vi "Efficiency Math.vi"(4 "SMU 2 Current Measurements":dbl[](array[numeric]), 5 "SMU 1 Voltage Measurements":dbl[](array[numeric]), 6 "SMU 2 Voltage Measurements":dbl[](array[numeric]), 7 "SMU 1 Current Measurements":dbl[](array[numeric]), 9 "# Voltage Divisions":i32, 10 "# Points":i32, 11 "XYGraph in":refnum<vi>) -> (3 "Array":cluster{"Array":dbl[], "Array":dbl[]}[](array[cluster]))   [LabVIEW 2014]
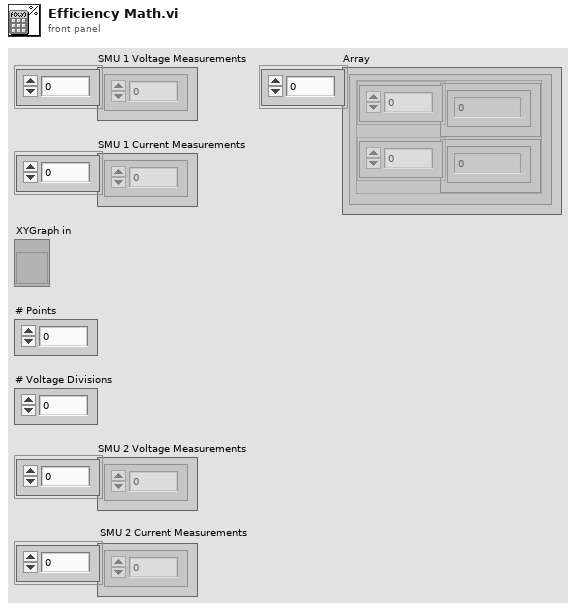
[diagram p1: front panel]
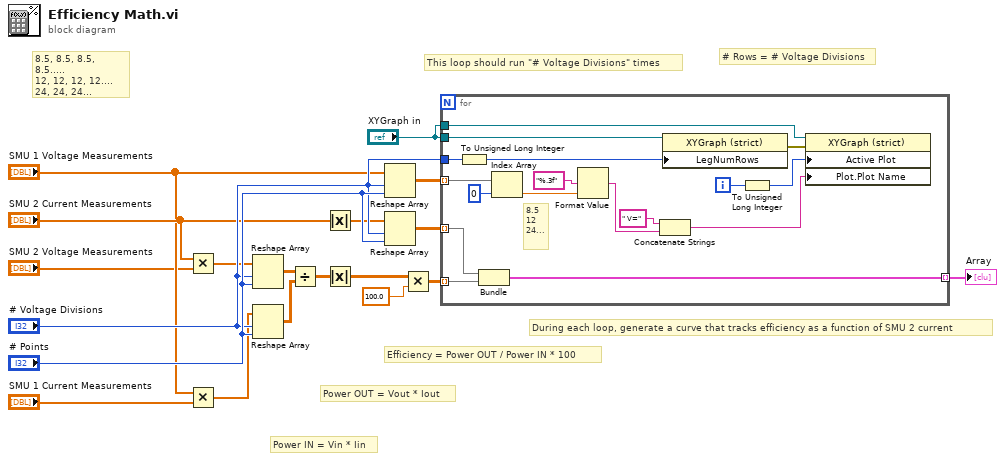
[diagram p0: block diagram]
diagram:
  # "Efficiency = Power OUT / Power IN * 100"
  # "# Rows = # Voltage Divisions"
  # "8.5, 8.5, 8.5, 8.5.....\n12, 12, 12, 12....\n24, 24, 24..."
  # "This loop should run \"# Voltage Divisions\" times"
  # "During each loop, generate a curve that tracks efficiency as a function of SMU 2 current"
  # "Power IN = Vin * Iin"
  # "Power OUT = Vout * Iout"
  n1 = Multiply(x="SMU 2 Current Measurements", y="SMU 2 Voltage Measurements") -> (x*y=w6:dbl[])
  n2 = Multiply(x="SMU 1 Voltage Measurements", y="SMU 1 Current Measurements") -> (x*y=w5:dbl[])
  n3 = Reshape Array(w6, "# Voltage Divisions", "# Points") -> (w7:dbl[][])
  n4 = Reshape Array(w5, "# Voltage Divisions", "# Points") -> (w8:dbl[][])
  n5 = Divide(x=w7, y=w8) -> (x/y=w12:dbl[][])
  n6 = Absolute Value(x="SMU 2 Current Measurements") -> (abs(x)=w14:dbl[])
  n7 = Absolute Value(x=w12) -> (abs(x)=w18:dbl[][])
  n8 = Reshape Array("SMU 1 Voltage Measurements", "# Voltage Divisions", "# Points") -> (w11:dbl[][])
  n9 = Reshape Array(w14, "# Voltage Divisions", "# Points") -> (w9:dbl[][])
  n10 = Multiply(x=w18, y=100.0) -> (x*y=w19:dbl[][])
  n11 = for {
    tunnel: w9 -> [w36] mode=indexing
    tunnel: w19 -> [w35] mode=indexing
    tunnel: [w34] -> w10 mode=indexing
    tunnel: "# Voltage Divisions" -> [w22]
    tunnel: w11 -> [w27] mode=indexing
    tunnel: "XYGraph in" -> [w25]
    tunnel: "XYGraph in" -> [w24]
    i -> [w21]
    # "8.5\n12\n24..."
    n12 = To Unsigned Long Integer(number=w22) -> (unsigned 32bit integer=w23:u32)
    n13 = Bundle(w36, w35) -> (w34:cluster{dbl[], dbl[]})  [unwired: 1 in]
    n14 = Index Array(array=w27, index=0) -> (element=w26:dbl)
    n15 = Format Value(format string="%.3f", value (0)=w26) -> (output string=w33:string)  [unwired: 1 out]
    n16 = Concatenate Strings(" V=" ("string"), w33) -> (w30:string)
    n17 = property on="Property Node" class="XYGraph (strict)"(reference=w25, "LegNumRows"=w23) -> (error out=w29:errorcluster)  [unwired: 1 in, 1 out]
    n18 = To Unsigned Long Integer(number=w21) -> (unsigned 32bit integer=w20:u32)
    n19 = property on="Property Node" class="XYGraph (strict)"(reference=w24, error in=w29, "Active Plot"=w20, "Plot.Plot Name"=w30) -> ()  [unwired: 2 out]
  }
  "Array" <- w10
